vi "GetContainedLibraries.vi"(8 "error in (no error)":errorcluster, 10 "LibDataIn[]":T1[](array[typedef]), 11 "Library in":refnum<vi>) -> (0 "error out":errorcluster, 3 "LibDataOut[]":T1[](array[typedef]))   [LabVIEW 2021, in "Migrator.lvlib"]
uses:
  Migrator.lvlib
  controls/LibraryData.ctl
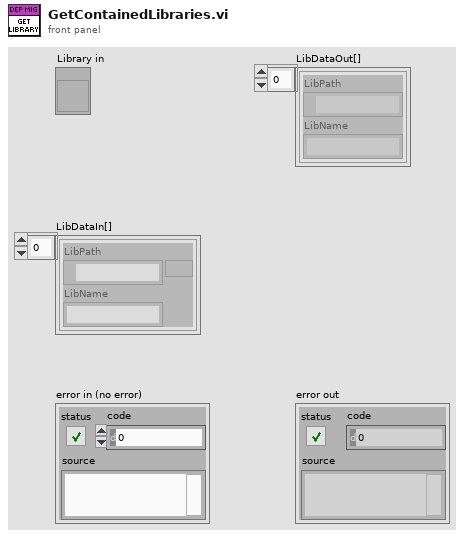
[diagram p1: front panel]
types:
  T1 = typedef "Migrator.lvlib/LibraryData.ctl" = cluster{"LibPath":path, "LibName":string}
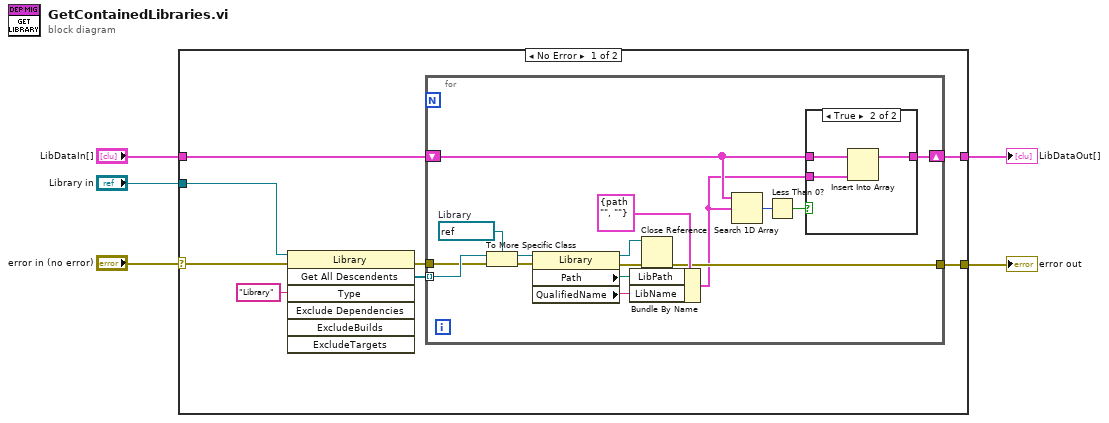
[diagram p0: block diagram]
diagram:
  n1 = case shown="No Error" "error in (no error)" {
    selector: "error in (no error)" -> [w12 w34]
    tunnel: [w13 w34] -> w5
    tunnel: "LibDataIn[]" -> [w11 _]
    tunnel: [w10 _] -> w2
    tunnel: "Library in" -> [w6 _]
    frame No Error {
      n2 = invoke class="Library" method="Get All Descendents"(reference=w6, error in=w12, "Type"="Library") -> (error out=w9:errorcluster, "All Descendents"=w8:refnum<vi>[])  [unwired: 4 in, 5 out]
      n3 = for {
        tunnel: w8 -> [w29] mode=indexing
        tunnel: w9 -> [w27]
        shift-right: [w24] -> w10
        shift-left: w11 -> [w16]
        tunnel: [w19] -> w13
        w25 = refnum<vi> refnum  # Library
        n4 = To More Specific Class(target class=w25, reference=w29, error in=w27) -> (specific class reference=w28:refnum<vi>, error out=w26:errorcluster)
        n5 = property class="Library"(reference=w28, error in=w26) -> (reference out=w18:refnum<vi>, error out=w20:errorcluster, "Path"=w22:path, "QualifiedName"=w21:string)
        n6 = Bundle By Name(cluster=T1 {"LibPath"=path "", "LibName"=""}, "LibPath"=w22, "LibName"=w21) -> (w15:T1)
        n7 = Close Reference(reference=w18, error in (no error)=w20) -> (error out=w19:errorcluster)
        n8 = Search 1D Array(1D array=w16, element=w15) -> (index of element=w17:i32)  [unwired: 1 in]
        n9 = Less Than 0?(x=w17) -> (x < 0?=w14:bool)
        n10 = case shown="True" w14 {
          tunnel: [w30 w33] -> w24
          tunnel: w16 -> [w30 w32]
          tunnel: w15 -> [_ w31]
          frame False {
          }
          frame True {
            n11 = Insert Into Array(array=w32, new element=w31) -> (w33:T1[])  [unwired: 1 in]
          }
        }
      }
    }
    frame Error {
    }
  }
  "error out" <- w5
  "LibDataOut[]" <- w2
